vi "Programer.vi"(7 "ID":T1, 8 "error in":errorcluster, 9 "config path":path=path "C:/4.9.12.6034", 11 "Commands":string[][](array[string])) -> (0 "error out":errorcluster, 1 "error?":bool, 3 "Response":string)   [LabVIEW 2021]
uses:
  ID.ctl
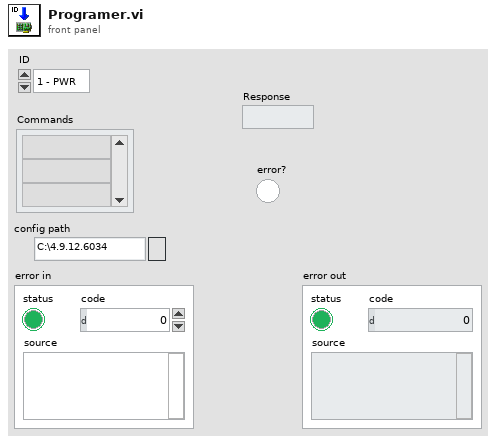
[diagram p1: front panel]
types:
  T1 = typedef "ID.ctl" = enum16{"1 - PWR", "2 - SM", "3 - DC", "4 - DM", "5 - WS", "6 - DS", "7 - WC", "8 - WA", "9 - WM", "10 - DA", "11 - WH", "12 - DH"}
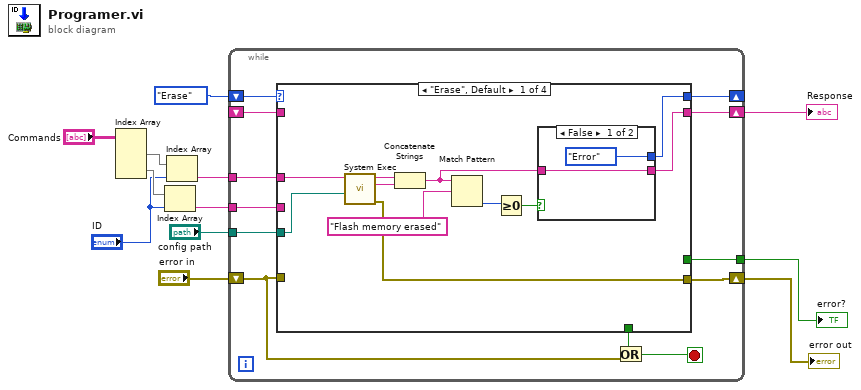
[diagram p0: block diagram]
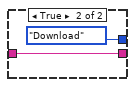
[diagram p2: hidden frame]
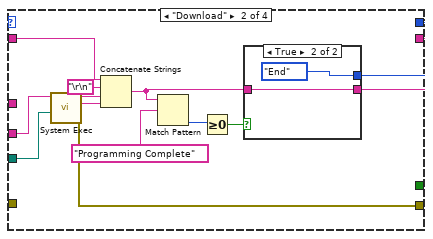
[diagram p3: hidden frame]
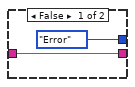
[diagram p4: hidden frame]
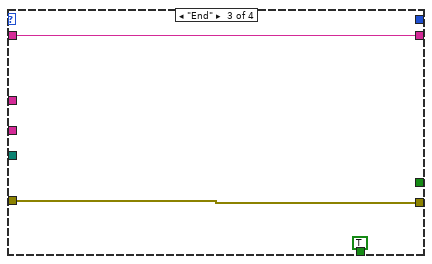
[diagram p5: hidden frame]
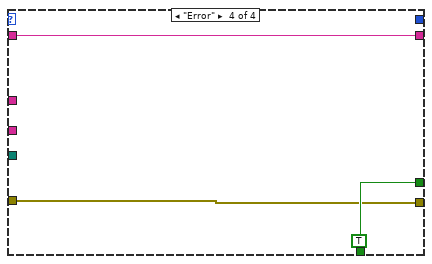
[diagram p6: hidden frame]
diagram:
  n1 = Index Array(array="Commands") -> (element #1=w10:string[], element #2=w9:string[])  [unwired: 4 in]
  n2 = Index Array(array=w9, index="ID") -> (element=w7:string)
  n3 = Index Array(array=w10, index="ID") -> (element=w6:string)
  n4 = while {
    shift-right: [w23] -> _
    shift-left: enum16{"Erase", "Download", "End", "Error"}."Erase" -> [w24]
    shift-right: [w22] -> w2
    shift-left: _ -> [w19]
    tunnel: w7 -> [w21]
    tunnel: w6 -> [w20]
    tunnel: [w18] -> w5
    shift-right: [w14] -> w3
    shift-left: "error in" -> [w15]
    tunnel: "config path" -> [w13]
    stop <- w17 stop-if-true
    n5 = case shown="\"Erase\", Default" w24 {
      tunnel: [w30 w42 _ _] -> w23
      tunnel: [w28 w43 w59 w60] -> w22
      tunnel: w21 -> [_ w46 _ _]
      tunnel: w20 -> [w27 _ _ _]
      tunnel: w19 -> [_ w44 w59 w60]
      tunnel: [_ _ TRUE w62] -> w16
      tunnel: [_ _ _ w62] -> w18
      tunnel: w15 -> [_ _ w57 w61]
      tunnel: [w26 w41 w57 w61] -> w14
      tunnel: w13 -> [w25 w40 _ _]
      frame "Erase", Default {
        n6 = call <vilib>:"System Exec.vi"("working directory"=w25, "command line"=w27) -> ("error out"=w26:errorcluster, "standard error"=w34:string, "standard output"=w35:string)  [unwired: 6 in, 1 out]
        n7 = Concatenate Strings(w35, w34) -> (w29:string)
        n8 = Match Pattern(string=w29, regular expression="Flash memory erased") -> (offset past match=w33:i32)  [unwired: 1 in, 3 out]
        n9 = Greater Or Equal To 0?(x=w33) -> (x >= 0?=w31:bool)
        n10 = case shown="False" w31 {
          tunnel: [enum16{"Erase", "Download", "End", "Error"}."Error" enum16{"Erase", "Download", "End", "Error"}."Download"] -> w30
          tunnel: w29 -> [w36 w38]
          tunnel: [w36 w38] -> w28
          frame False {
          }
          frame True {
          }
        }
      }
      frame "Download" {
        n11 = call <vilib>:"System Exec.vi"("working directory"=w40, "command line"=w46) -> ("error out"=w41:errorcluster, "standard error"=w51:string, "standard output"=w52:string)  [unwired: 6 in, 1 out]
        n12 = Concatenate Strings(w44, "\r\n", w52, w51) -> (w47:string)
        n13 = Match Pattern(string=w47, regular expression="Programming Complete") -> (offset past match=w50:i32)  [unwired: 1 in, 3 out]
        n14 = Greater Or Equal To 0?(x=w50) -> (x >= 0?=w48:bool)
        n15 = case shown="True" w48 {
          tunnel: [enum16{"Erase", "Download", "End", "Error"}."Error" enum16{"Erase", "Download", "End", "Error"}."End"] -> w42
          tunnel: w47 -> [w53 w55]
          tunnel: [w53 w55] -> w43
          frame False {
          }
          frame True {
          }
        }
      }
      frame "End" {
      }
      frame "Error" {
        w62 = TRUE
      }
    }
    n16 = Or(x=w16, y=w15) -> (x .or. y?=w17:bool)
  }
  "error?" <- w5
  "error out" <- w3
  "Response" <- w2
